vi "Sample TEMPLATE - READ.vi"() -> ()   [LabVIEW 2020, in "WaveFile.lvclass"]
uses:
  WaveFile.lvclass
  API/GSwFormDSP_class/GSwFormDSP.lvclass
panel:
  out "error out":errorcluster
  out "Time Data - READ":waveform(dbl)[](graph)
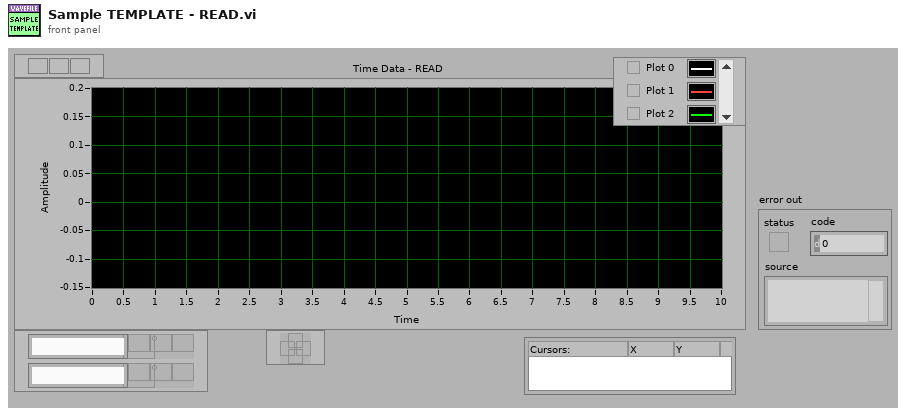
[diagram p1: front panel]
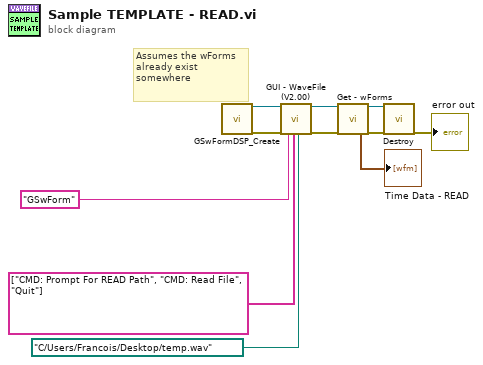
[diagram p0: block diagram]
diagram:
  # "Assumes the wForms already exist somewhere"
  n1 = call "GSwFormDSP_Create.vi"() -> ("reference out"=w4:refnum<class "GSwFormDSP.lvclass">, "error out"=w10:errorcluster)  [unwired: 18 in]
  n2 = call "GUI - WaveFile (V2.00).vi"("Time Data IN"=w4, "error in (no error)"=w10, "Application Name"="GSwForm", "State Queue"=string[] ["CMD: Prompt For READ Path", "CMD: Read File", "Quit"], "Wave - READ"=path "C:/Users/Francois/Desktop/temp.wav" ("Wave File Path - READ")) -> ("SubVI Time Data DUP"=w3:refnum<class "GSwFormDSP.lvclass">, "error out"=w7:errorcluster)  [unwired: 13 in]
  n3 = call-dynamic "Get - wForms.vi"("reference in"=w3, "error in (no error)"=w7) -> ("wForms"=→"Time Data - READ":waveform(dbl)[], "reference out"=w6:refnum<class "GSwFormDSP.lvclass">, "error out"=w5:errorcluster)  [unwired: 14 in, 1 out]
  n4 = call-dynamic "Destroy.vi"("reference in"=w6, "error in (no error)"=w5) -> ("error out"=→"error out":errorcluster)  [unwired: 16 in, 1 out]
